vi "get_info_sheet.vi"(3 "input_machine_reference.lvclass":refnum<class "machine.lvclass">) -> (0 "info_sheet_out":string, 1 "output_machine_reference.lvclass":refnum<class "machine.lvclass">)   [LabVIEW 2014, in "machine.lvclass"]
uses:
  machine.lvclass
  machine.lvclass/machine.ctl
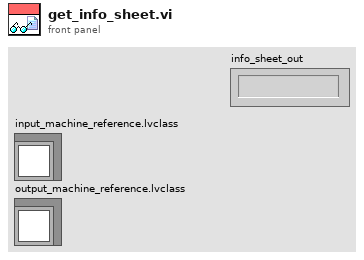
[diagram p1: front panel]
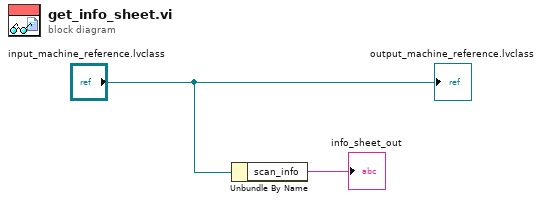
[diagram p0: block diagram]
diagram:
  n1 = Unbundle By Name("input_machine_reference.lvclass") -> ("scan_info"=→"info_sheet_out":string)
  "output_machine_reference.lvclass" <- "input_machine_reference.lvclass"
